vi "Test Operations.vi"(11 "Error in":errorcluster) -> (15 "Error out":errorcluster)   [LabVIEW 2020, in "LogicalComparisonTest.lvlib"]
doc: "This VI is the validating VI for the Logical comparison"
uses:
  LogicalComparisonTest.lvlib
  <vilib>/addons/_JKI Toolkits/Caraya/classes/Test Suite/Define Test Suite (JUnit Report).vi
  <vilib>/SLL Drona/APIs/Stimulus/ControlValue/SetValueAuto.vi
  <vilib>/SLL Drona/APIs/Assert/AssertControlValue/Equal.vi
  <vilib>/SLL Drona/APIs/Stimulus/VI/CloseVI.vi
  <vilib>/Utility/error.llb/Error Cluster From Error Code.vi
  <vilib>/ErrorRing/Error Ring.xnode
  <vilib>/addons/_JKI Toolkits/Caraya/classes/Test Suite/Test Suite.lvclass
  <vilib>/SLL Drona/Drona.lvlib
  <vilib>/addons/_JKI Toolkits/Caraya/classes/Test/Test.lvclass
  <vilib>/SLL Drona/APIs/Stimulus/ControlValue/ControlValue.lvlib
  <vilib>/SLL Drona/APIs/Assert/AssertControlValue/AssertControlValue.lvlib
  <vilib>/Wiresmith Technology/G CLI/CLI Class/CLI.lvclass
  <vilib>/SLL Drona/APIs/Stimulus/VI/VI.lvlib
panel:
  # "LOGICAL COMPARISION TEST"
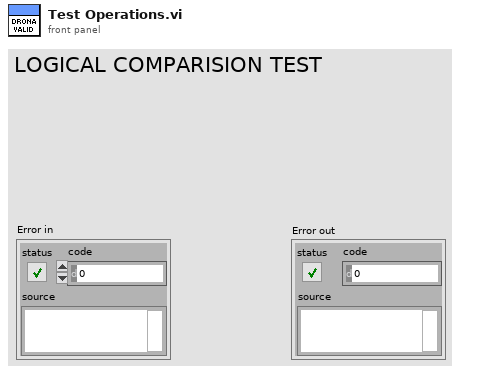
[diagram p1: front panel]
types:
  T1 = cluster{"A":dbl, "B":dbl, "Operations":enum16{"A>B", "A<B", "A>=B", "A<=B", "A=B", "A!=B"}, "Result":bool}[]
  T2 = enum16{"A>B", "A<B", "A>=B", "A<=B", "A=B", "A!=B"}
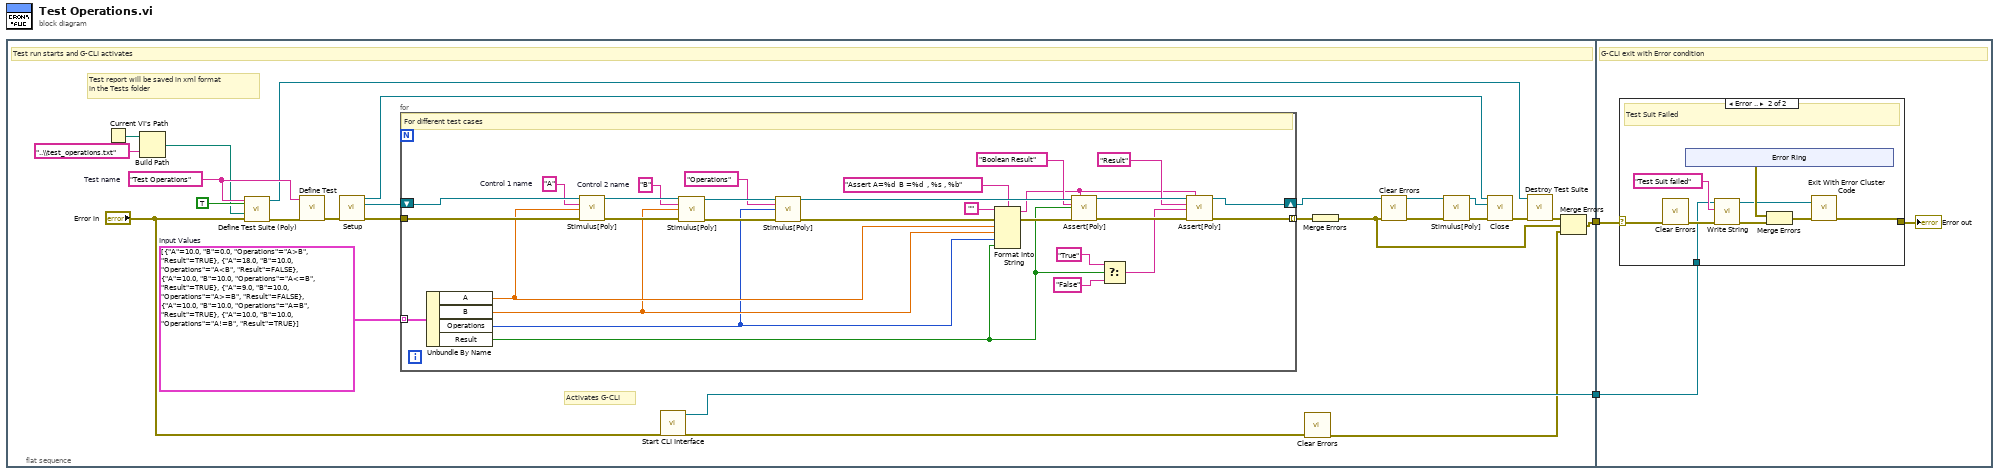
[diagram p0: block diagram]
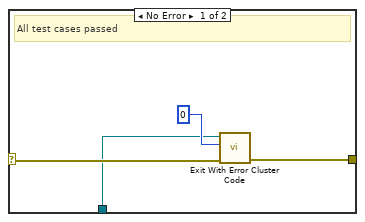
[diagram p2: hidden frame]
diagram:
  n1 = flat-sequence {
    tunnel: [w18] -> w2
    tunnel: [w16] -> w1
    tunnel: w2 -> [w59]
    tunnel: w1 -> [w57]
    frame #0 {
      w13 = "Test Operations"  # Test name
      w24 = T1 [{"A"=10.0, "B"=0.0, "Operations"=enum."A>B", "Result"=TRUE}, {"A"=18.0, "B"=10.0, "Operations"=enum."A<B", "Result"=FALSE}, {"A"=10.0, "B"=10.0, "Operations"=enum."A<=B", "Result"=TRUE}, {"A"=9.0, "B"=10.0, "Operations"=enum."A>=B", "Result"=FALSE}, {"A"=10.0, "B"=10.0, "Operations"=enum."A=B", "Result"=TRUE}, {"A"=10.0, "B"=10.0, "Operations"=enum."A!=B", "Result"=TRUE}]  # Input Values
      # "Test report will be saved in xml format\nin the Tests folder"
      # "Activates G-CLI"
      # "Test run starts and G-CLI activates"
      n2 = Current VI's Path() -> (path=w11:path)
      n3 = Build Path(base path=w11, name or relative path="..\\test_operations.txt") -> (appended path=w9:path)
      n4 = call-poly <vilib>:"Define Test Suite (Poly).vi"("error in (no error)"="Error in", "Report Path"=w9, "Interactive"=TRUE, "Label (VI Title)"=w13) -> ("error out"=w15:errorcluster, "Test Suite"=w6:refnum<class "Test Suite.lvclass">)  [unwired: 5 in, 1 out]
      n5 = call <vilib>:"Define Test.vi"("error in (no error)"=w15, "Label (VI Title)"=w13) -> ("error out"=w27:errorcluster)  [unwired: 8 in, 1 out]
      n6 = call <vilib>:"Setup.vi"("error in"=w27) -> ("Application Ref"=w23:refnum<vi>, "VI Reference Out"=w25:refnum<vi>, "error out"=w26:errorcluster)  [unwired: 12 in]
      n7 = for {
        shift-right: [w40] -> w22
        shift-left: w25 -> [w53]
        tunnel: w24 -> [w50] mode=indexing
        tunnel: w26 -> [w56]
        tunnel: [w28] -> w19 mode=indexing
        w47 = "B"  # Control 2 name
        w49 = "A"  # Control 1 name
        # "For different test cases"
        n8 = Unbundle By Name(w50) -> ("A"=w32:dbl, "B"=w31:dbl, "Operations"=w30:T2, "Result"=w29:bool)
        n9 = call-poly <vilib>:"Stimulus[Poly].vi"("VI Reference In"=w53, "Control Path"=w49, "Value (Signaling)"=w32, "error in"=w56) -> ("VI Reference Out"=w48:refnum<vi>, "error out"=w55:errorcluster)  [unwired: 10 in]
        n10 = call-poly <vilib>:"Stimulus[Poly].vi"("VI Reference In"=w48, "Control Path"=w47, "Value (Signaling)"=w31, "error in"=w55) -> ("VI Reference Out"=w46:refnum<vi>, "error out"=w54:errorcluster)  [unwired: 10 in]
        n11 = call-poly <vilib>:"Stimulus[Poly].vi"("VI Reference In"=w46, "Control Path"="Operations", "Value (Signaling)"=w30, "error in"=w54) -> ("VI Reference Out"=w44:refnum<vi>, "error out"=w52:errorcluster)  [unwired: 10 in]
        n12 = Format Into String(format string="Assert A=%d  B =%d  , %s , %b", initial string="", error in=w52, w32, w31, w30, w29) -> (resulting string=w38:string, error out=w51:errorcluster)
        n13 = call-poly <vilib>:"Assert[Poly].vi"("VI Reference In"=w44, "Test Label"=w38, "Control Path"="Boolean Result", "Control Value"=w29, "Error In"=w51) -> ("VI Reference Out"=w41:refnum<vi>, "Error Out"=w42:errorcluster)  [unwired: 9 in]
        n14 = Select(t="True", s=w29, f="False") -> (s? t:f=w33:string)
        n15 = call-poly <vilib>:"Assert[Poly].vi"("VI Reference In"=w41, "Test Label"=w38, "Control Path"="Result", "Control Value"=w33, "Error In"=w42) -> ("VI Reference Out"=w40:refnum<vi>, "Error Out"=w28:errorcluster)  [unwired: 9 in]
      }
      n16 = call <vilib>:"Start CLI Interface.vi"("error in (no error)"="Error in") -> ("error out"=w17:errorcluster, "CLI out"=w16:refnum<class "CLI.lvclass">)  [unwired: 7 in, 2 out]
      n17 = call <vilib>:"Clear Errors.vi"("error in (no error)"=w17) -> ("error out"=w3:errorcluster)  [unwired: 5 in, 1 out]
      n18 = Merge Errors(w19) -> (w4:errorcluster)
      n19 = call <vilib>:"Clear Errors.vi"("error in (no error)"=w4) -> ("error out"=w5:errorcluster)  [unwired: 5 in, 1 out]
      n20 = call-poly <vilib>:"Stimulus[Poly].vi"("VI Reference In"=w22, "error in"=w5) -> ("VI Reference Out"=w20:refnum<vi>, "error out"=w21:errorcluster)  [unwired: 12 in]
      n21 = call <vilib>:"Close.vi"("Application Ref"=w23, "VI Reference"=w20, "error in"=w21) -> ("error out"=w8:errorcluster)  [unwired: 12 in]
      n22 = call-dynamic "Destroy Test Suite.vi"("error in (no error)"=w8, "Test Suite in"=w6) -> ("error out"=w7:errorcluster)  [unwired: 8 in, 1 out]
      n23 = Merge Errors(w7, w4, w3) -> (w18:errorcluster)
    }
    frame #1 {
      # "G-CLI exit with Error condition"
      n24 = case shown="Error .." w59 {
        selector: w59 -> [w63 w70]
        tunnel: w57 -> [w61 w65]
        tunnel: [w60 w72] -> w58
        frame No Error {
          # "All test cases passed"
          n25 = call <vilib>:"Exit With Error Cluster Code.vi"("error in (no error)"=w63, "No Error Code (0)"=0, "CLI in"=w61) -> ("error out"=w60:errorcluster)  [unwired: 8 in]
        }
        frame Error {
          # "Test Suit Failed"
          n26 = call <vilib>:"Clear Errors.vi"("error in (no error)"=w70) -> ("error out"=w69:errorcluster)  [unwired: 5 in, 1 out]
          n27 = xnode "Error Ring"() -> ("error out"=w68:errorcluster)
          n28 = call <vilib>:"Write String.vi"("error in (no error)"=w69, "Text to Write"="Test Suit failed", "CLI in"=w65) -> ("error out"=w67:errorcluster, "CLI out"=w64:refnum<class "CLI.lvclass">)  [unwired: 7 in]
          n29 = Merge Errors(w68, w67) -> (w66:errorcluster)
          n30 = call <vilib>:"Exit With Error Cluster Code.vi"("error in (no error)"=w66, "CLI in"=w64) -> ("error out"=w72:errorcluster)  [unwired: 9 in]
        }
      }
      "Error out" <- w58
    }
  }
